vi "AG34980A_Configure_Resistance.vi"(0 "VISA resource name":refnum<visa-resource-name>, 5 "Range (7:Auto)":T2(ring)=enum."Auto", 7 "Resolution (5:Default)":T1(ring)=enum."Default", 9 "Autozero (0:ON)":enum16{"On", "Off", "Once"}(ring), 11 "error in (no error)":errorcluster, 12 "Offset Compensation (F:Off)":bool) -> (4 "VISA resource name out":refnum<visa-resource-name>, 15 "error out":errorcluster)   [LabVIEW 2022 SP3, in "DMM_Keysight_34980A.lvlib" / "DMM_Keysight_34980A.lvclass"]
doc: "This VI allows you to control various settings for performing resistance measurements. You can independently control the range, resolution, autozero mode, and offset compensation settings."
uses:
  DMM_Keysight_34980A.lvclass
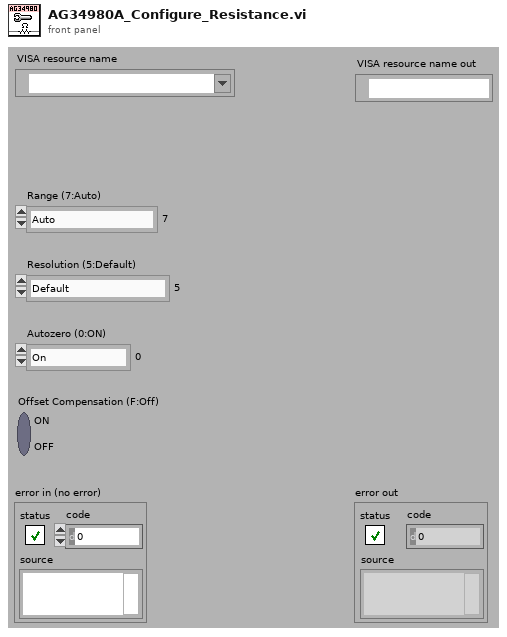
[diagram p1: front panel]
types:
  T1 = enum16{"4 1/2", "5 1/2", "6 1/2", "Least", "Highest", "Default"}
  T2 = enum16{"100 Ohm", "1 kOhm", "10 kOhm", "100 kOhm", "1 MOhm", "10 MOhm", "100 MOhm", "Auto", "Minimum", "Maximum"}
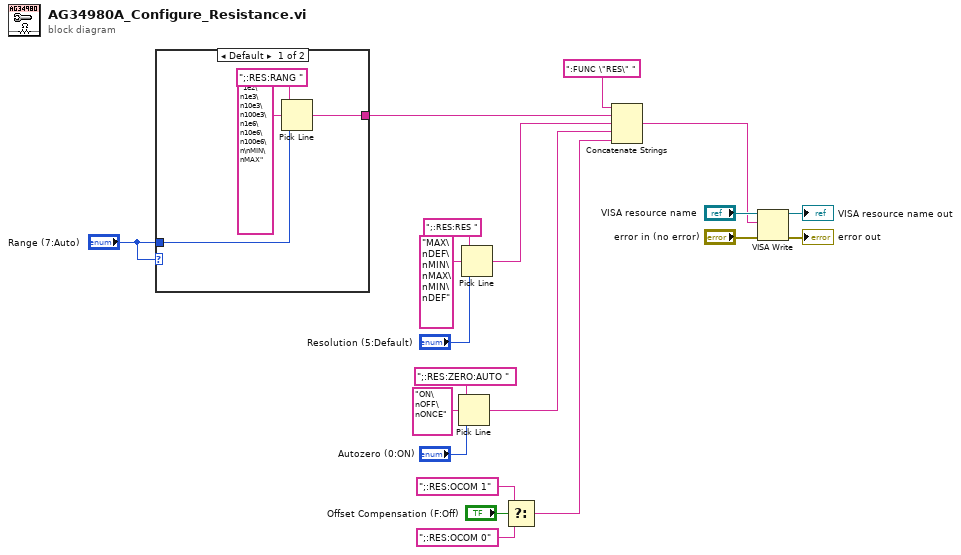
[diagram p0: block diagram]
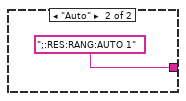
[diagram p2: hidden frame]
diagram:
  n1 = case shown="Default" "Range (7:Auto)" {
    tunnel: "Range (7:Auto)" -> [w23 _]
    tunnel: [w22 ";:RES:RANG:AUTO 1"] -> w19
    frame Default {
      n2 = Pick Line(string ("")=";:RES:RANG ", multi-line string="1e2\n1e3\n10e3\n100e3\n1e6\n10e6\n100e6\n\nMIN\nMAX", line index=w23) -> (output string=w22:string)
    }
    frame "Auto" {
    }
  }
  n3 = Pick Line(string ("")=";:RES:ZERO:AUTO ", multi-line string="ON\nOFF\nONCE", line index="Autozero (0:ON)") -> (output string=w8:string)
  n4 = Pick Line(string ("")=";:RES:RES ", multi-line string="MAX\nDEF\nMIN\nMAX\nMIN\nDEF", line index="Resolution (5:Default)") -> (output string=w1:string)
  n5 = Select(t=";:RES:OCOM 1", s="Offset Compensation (F:Off)", f=";:RES:OCOM 0") -> (s? t:f=w7:string)
  n6 = Concatenate Strings(":FUNC \"RES\" ", w19, w1, w8, w7) -> (w13:string)
  n7 = VISA Write(VISA resource name="VISA resource name", write buffer=w13, error in (no error)="error in (no error)") -> (VISA resource name out=→"VISA resource name out":refnum<visa-resource-name>, error out=→"error out":errorcluster)  [unwired: 1 out]
